vi "Split Quoted String.vi"(9 "delimiters (\\s,\\t,\\r,\\n)":string[](array[string])=[" ", "\t", "\r", "\n"], 10 "quotes (\",',`)":string[](array[string])=["\"", "'", "`"], 11 "quoted string":string) -> (2 "quote type":string[](array[string]), 3 "elements":string[](array[string]))   [LabVIEW 2019]
doc: "<b>Description</b> This VI splits a quoted string into an array of strings using the specified delimeters. This is suitable for splitting typical command-style strings into individual arguments or for splitting CSV data containing quoted strings.\n\nThis VI splits a quoted string into individual elements.\n\n<b>Inputs</b>\n<b>quoted string</b>: A string containing quoted and/or unquoted elements.\n<b>quotes </b>: (\"',',`)\nA list of allowable quote characters.\n<b>delimiters </b>: (\\s,\\t,\\r,\\n)\nA list of delimeters between string elements. Add ',' to this list to split comma-separated values.\n\n\n<b>Outputs</b>\n<b>quote type</b>: The quote character used to delimit elements in the input string. Empty strings in this output indicate that the particular element was unquoted.\n<b>elements</b>: Elements of the original string."
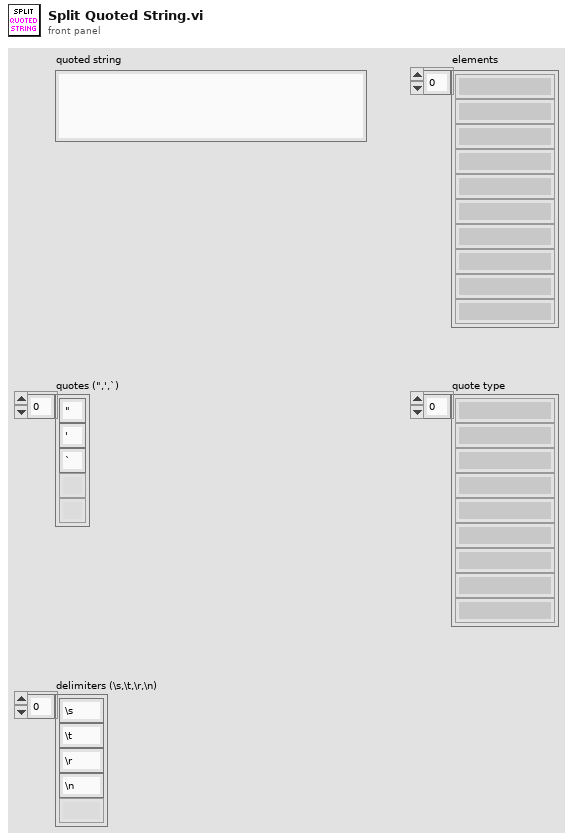
[diagram p1: front panel]
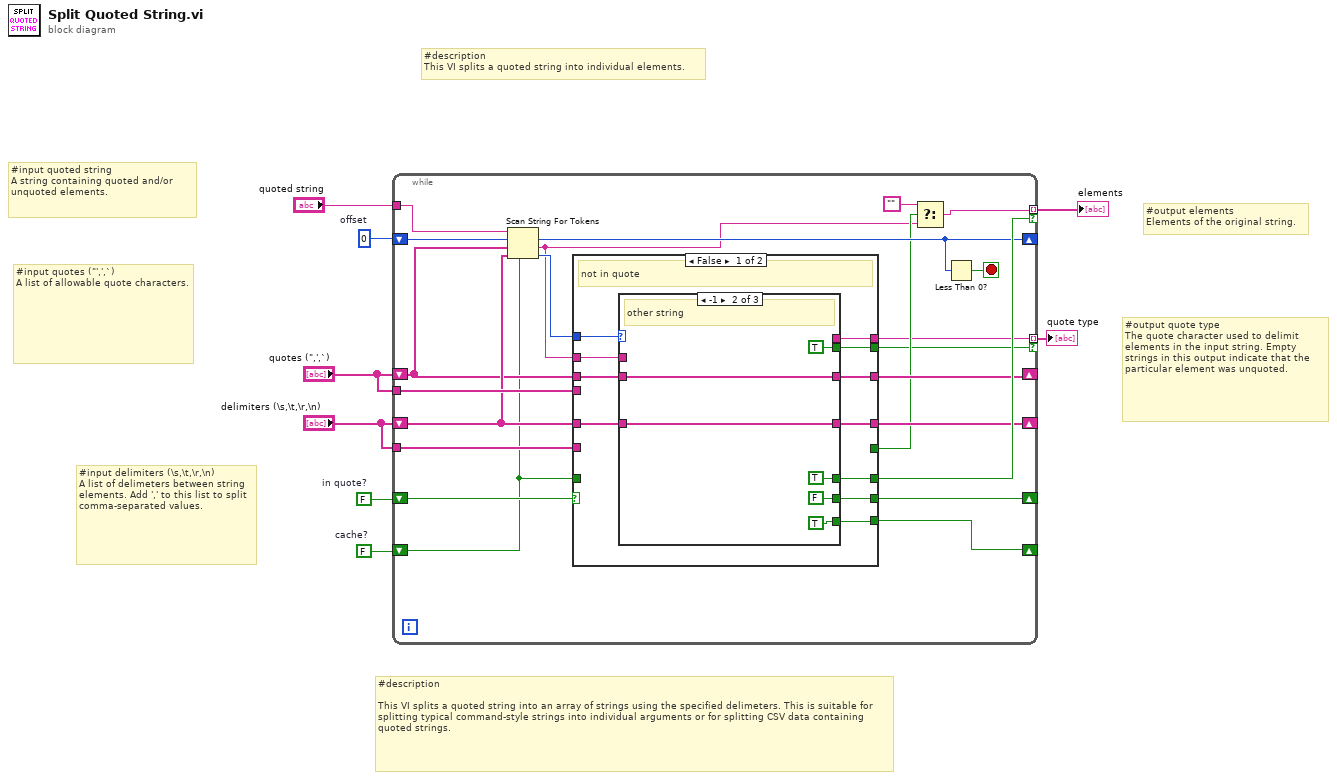
[diagram p0: block diagram]
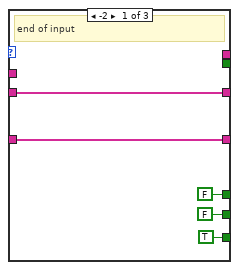
[diagram p2: hidden frame]
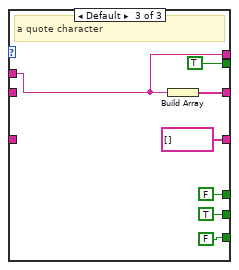
[diagram p3: hidden frame]
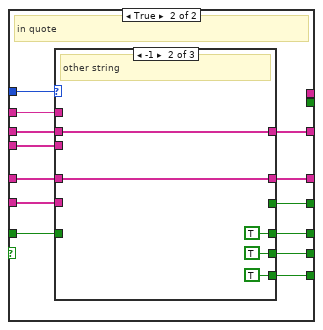
[diagram p4: hidden frame]
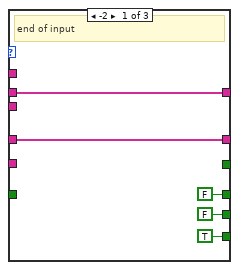
[diagram p5: hidden frame]
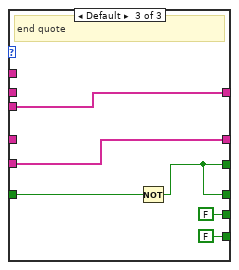
[diagram p6: hidden frame]
diagram:
  w2 = FALSE  # cache?
  w6 = FALSE  # in quote?
  w7 = 0  # offset
  # "#output quote type\nThe quote character used to delimit elements in the input string. Empty strings in this output indicate that the particular element was unquoted."
  # "#output elements\nElements of the original string."
  # "#input quoted string\nA string containing quoted and/or unquoted elements."
  # "#input quotes (\"',',`)\nA list of allowable quote characters."
  # "#input delimiters (\\s,\\t,\\r,\\n)\nA list of delimeters between string elements. Add ',' to this list to split comma-separated values."
  # "#description \n\nThis VI splits a quoted string into an array of strings using the specified delimeters. This is suitable for splitting typical command-style strings into individual arguments or for splitting CSV data containing quoted strings."
  # "#description\nThis VI splits a quoted string into individual elements."
  n1 = while {
    tunnel: "quoted string" -> [w30]
    shift-right: [w20] -> _
    shift-left: w7 -> [w29]
    shift-right: [w10] -> _
    shift-left: w6 -> [w28]
    shift-right: [w24] -> _
    shift-left: "quotes (\",',`)" -> [w18]
    shift-right: [w23] -> _
    shift-left: "delimiters (\\s,\\t,\\r,\\n)" -> [w22]
    tunnel: [w12] -> w5 mode=indexing if=w27
    tunnel: "quotes (\",',`)" -> [w26]
    tunnel: "delimiters (\\s,\\t,\\r,\\n)" -> [w25]
    shift-right: [w17] -> _
    shift-left: w2 -> [w16]
    tunnel: [w11] -> w1 mode=indexing if=w9
    stop <- w21 stop-if-true
    n2 = Scan String For Tokens(4:w16, 6:w22, 7:w18, 8:w29, 9:w30) -> (0:w19:i32, 1:w14:string, 2:w20:i32)  [unwired: 1 in, 1 out]
    n3 = case shown="False" w28 {
      tunnel: w19 -> [w41 w72]
      tunnel: [w40 w71] -> w27
      tunnel: [w39 w70] -> w10
      tunnel: w14 -> [w38 w69]
      tunnel: w26 -> [_ w64]
      tunnel: w25 -> [_ w63]
      tunnel: [w37 w68] -> w24
      tunnel: w18 -> [w36 w67]
      tunnel: [w35 w66] -> w23
      tunnel: w22 -> [w34 w65]
      tunnel: [w33 w62] -> w17
      tunnel: w16 -> [_ w61]
      tunnel: [_ w60] -> w15
      tunnel: [w32 _] -> w11
      tunnel: [w31 _] -> w9
      frame False {
        # "not in quote"
        n4 = case shown="-1" w41 {
          tunnel: [FALSE TRUE FALSE] -> w40
          tunnel: [FALSE FALSE TRUE] -> w39
          tunnel: w38 -> [_ _ w54]
          tunnel: [w44 w50 w57] -> w37
          tunnel: w36 -> [w44 w50 _]
          tunnel: [w43 w49 string[] [] ("delimiters (\\s,\\t,\\r,\\n)")] -> w35
          tunnel: w34 -> [w43 w49 _]
          tunnel: [TRUE TRUE FALSE] -> w33
          tunnel: [_ _ w54] -> w32
          tunnel: [_ TRUE TRUE] -> w31
          frame -2 {
            # "end of input"
          }
          frame -1 {
            # "other string"
          }
          frame Default {
            # "a quote character"
            n5 = Build Array(w54) -> (w57:string[])
          }
        }
      }
      frame True {
        # "in quote"
        n6 = case shown="-1" w72 {
          tunnel: [FALSE TRUE w83] -> w71
          tunnel: [FALSE TRUE FALSE] -> w70
          tunnel: w69 -> [_ _ _]
          tunnel: [w75 w80 w87] -> w68
          tunnel: w67 -> [w75 w80 _]
          tunnel: [w74 w79 w86] -> w66
          tunnel: w65 -> [w74 w79 _]
          tunnel: w64 -> [_ _ w87]
          tunnel: w63 -> [_ _ w86]
          tunnel: [TRUE TRUE FALSE] -> w62
          tunnel: w61 -> [_ _ w84]
          tunnel: [_ _ w83] -> w60
          frame -2 {
            # "end of input"
          }
          frame -1 {
            # "other string"
          }
          frame Default {
            # "end quote"
            n7 = Not(x=w84) -> (.not. x?=w83:bool)
          }
        }
      }
    }
    n8 = Select(t="", s=w15, f=w14) -> (s? t:f=w12:string)
    n9 = Less Than 0?(x=w20) -> (x < 0?=w21:bool)
  }
  "elements" <- w5
  "quote type" <- w1
